vi "To Value.vi"(8 "error in (no error)":errorcluster, 10 "PV Data in":refnum<class "PV Data.lvclass">, 11 "NT Scalar (Numeric) in":refnum<class "NT Scalar (Numeric).lvclass">) -> (0 "error out":errorcluster, 2 "PV Data out":refnum<class "PV Data.lvclass">, 3 "NT Scalar (Numeric) out":refnum<class "NT Scalar (Numeric).lvclass">)   [LabVIEW 2020, in "PV Access.lvlib" / "PV Data.lvlib" / "NT Scalar (Numeric).lvclass"]
uses:
  NT Scalar (Numeric).lvclass
  NT Scalar (Numeric).lvclass/NT Scalar (Numeric).ctl
  PV Data/PV Data.lvclass
  PV Data/Write Field (Variant).vi
  NT Scalar/NT Scalar.lvclass
  PV Data/Write Field (String).vi
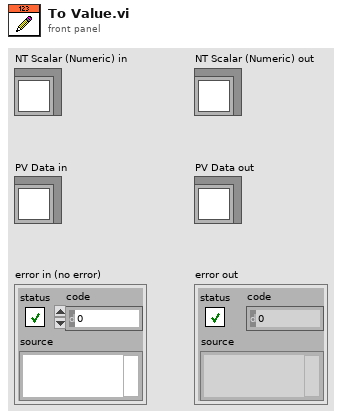
[diagram p1: front panel]
types:
  T1 = typedef "PV Access.lvlib/PV Data.lvlib/Alarm Limits.ctl" = cluster{"Active":bool, "Low Alarm Limit":variant, "Low Warning Limit":variant, "High Warning Limit":variant, "High Alarm Limit":variant, "Low Alarm Severity":T2, "Low Warning Severity":T2, "High Warning Severity ":T2, "High Alarm Severity":T2, "Hysteresis":dbl}
  T2 = typedef "PV Access.lvlib/PV Data.lvlib/Alarm Severity.ctl" = enum32{"no", "minor", "major", "record", "invalid", "undefined", ""}
  T3 = typedef "PV Access.lvlib/PV Data.lvlib/Display Form.ctl" = enum32{"Default", "String", "Binary", "Decimal", "Hex", "Exponential", "Engineering"}
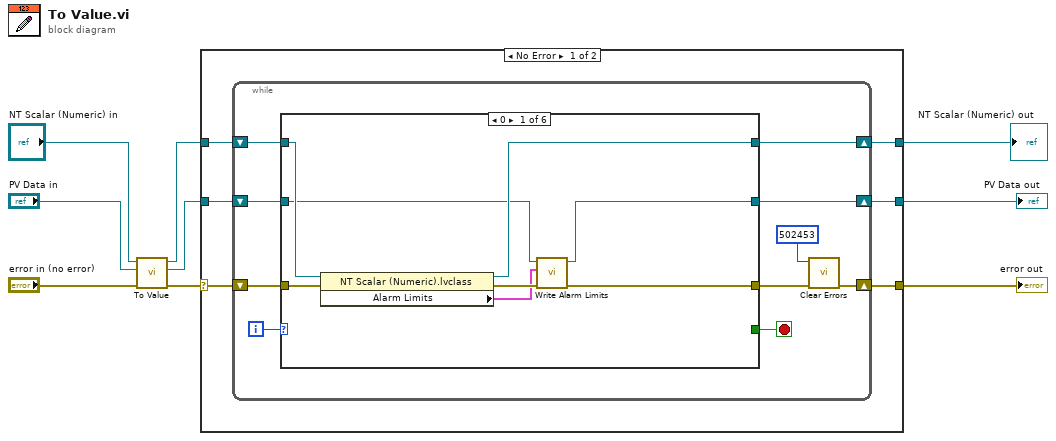
[diagram p0: block diagram]
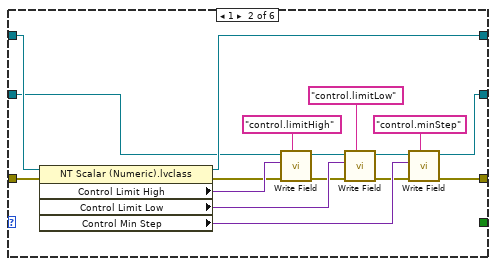
[diagram p2: hidden frame]
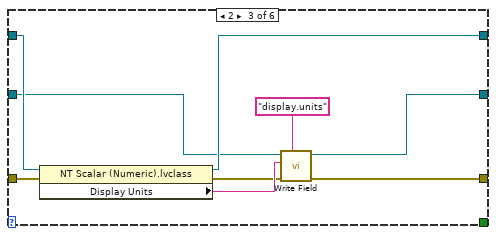
[diagram p3: hidden frame]
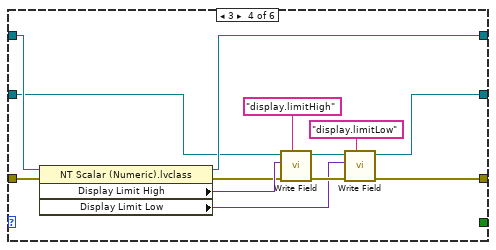
[diagram p4: hidden frame]
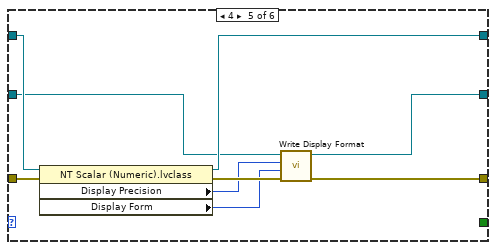
[diagram p5: hidden frame]
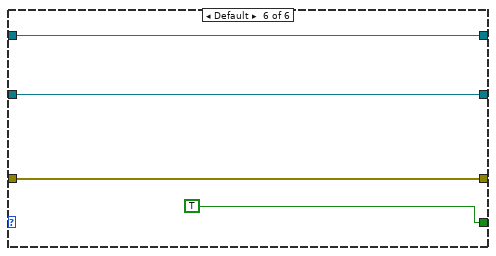
[diagram p6: hidden frame]
diagram:
  n1 = call-parent "To Value.vi"("error in (no error)"="error in (no error)", "PV Data in"="PV Data in", "NT Scalar in"="NT Scalar (Numeric) in") -> ("error out"=w5:errorcluster, "PV Data out"=w1:refnum<class "PV Data.lvclass">, "NT Scalar out"=w2:refnum<class "NT Scalar (Numeric).lvclass">)  [unwired: 6 in]
  n2 = case shown="No Error" w5 {
    selector: w5 -> [w15 w88]
    tunnel: [w12 w88] -> w7
    tunnel: [w10 w87] -> w9
    tunnel: w2 -> [w14 w87]
    tunnel: w1 -> [w13 w86]
    tunnel: [w11 w86] -> w8
    frame No Error {
      n3 = while {
        shift-right: [w19] -> w12
        shift-left: w15 -> [w24]
        shift-right: [w18] -> w11
        shift-left: w13 -> [w23]
        shift-right: [w17] -> w10
        shift-left: w14 -> [w22]
        i -> [w25]
        stop <- w16 stop-if-true
        n4 = case shown="0" w25 {
          tunnel: w24 -> [w33 w50 w59 w72 w81 w84]
          tunnel: w23 -> [w28 w39 w51 w62 w78 w83]
          tunnel: w22 -> [w32 w49 w58 w71 w80 w82]
          tunnel: [w26 w37 w54 w60 w76 w84] -> w20
          tunnel: [w27 w38 w55 w61 w77 w83] -> w18
          tunnel: [w31 w48 w57 w70 w79 w82] -> w17
          tunnel: [_ _ _ _ _ TRUE] -> w16
          frame 0 {
            n5 = property class="NT Scalar (Numeric).lvclass"(reference=w32, error in=w33) -> (reference out=w31:refnum<class "NT Scalar (Numeric).lvclass">, error out=w30:errorcluster, "Alarm Limits"=w29:T1)
            n6 = call "Write Alarm Limits.vi"("error in"=w30, "Alarm Limits"=w29, "PV Data in"=w28) -> ("error out"=w26:errorcluster, "PV Data out"=w27:refnum<class "PV Data.lvclass">)  [unwired: 7 in]
          }
          frame 1 {
            n7 = property class="NT Scalar (Numeric).lvclass"(reference=w49, error in=w50) -> (reference out=w48:refnum<class "NT Scalar (Numeric).lvclass">, error out=w44:errorcluster, "Control Limit High"=w47:variant, "Control Limit Low"=w46:variant, "Control Min Step"=w45:variant)
            n8 = call-poly "Write Field.vi"("field name"="control.limitHigh", "error in (no error)"=w44, "value in"=w47, "PV Data in"=w39) -> ("error out"=w43:errorcluster, "PV Data out"=w40:refnum<class "PV Data.lvclass">)  [unwired: 5 in, 1 out]
            n9 = call-poly "Write Field.vi"("field name"="control.limitLow", "error in (no error)"=w43, "value in"=w46, "PV Data in"=w40) -> ("error out"=w42:errorcluster, "PV Data out"=w41:refnum<class "PV Data.lvclass">)  [unwired: 5 in, 1 out]
            n10 = call-poly "Write Field.vi"("field name"="control.minStep", "error in (no error)"=w42, "value in"=w45, "PV Data in"=w41) -> ("error out"=w37:errorcluster, "PV Data out"=w38:refnum<class "PV Data.lvclass">)  [unwired: 5 in, 1 out]
          }
          frame 2 {
            n11 = property class="NT Scalar (Numeric).lvclass"(reference=w58, error in=w59) -> (reference out=w57:refnum<class "NT Scalar (Numeric).lvclass">, error out=w52:errorcluster, "Display Units"=w53:string)
            n12 = call-poly "Write Field.vi"("field name"="display.units", "error in"=w52, "value"=w53, "PV Data in"=w51) -> ("error out"=w54:errorcluster, "PV Data out"=w55:refnum<class "PV Data.lvclass">)  [unwired: 5 in, 1 out]
          }
          frame 3 {
            n13 = property class="NT Scalar (Numeric).lvclass"(reference=w71, error in=w72) -> (reference out=w70:refnum<class "NT Scalar (Numeric).lvclass">, error out=w63:errorcluster, "Display Limit High"=w65:variant, "Display Limit Low"=w64:variant)
            n14 = call-poly "Write Field.vi"("field name"="display.limitHigh", "error in (no error)"=w63, "value in"=w65, "PV Data in"=w62) -> ("error out"=w66:errorcluster, "PV Data out"=w67:refnum<class "PV Data.lvclass">)  [unwired: 5 in, 1 out]
            n15 = call-poly "Write Field.vi"("field name"="display.limitLow", "error in (no error)"=w66, "value in"=w64, "PV Data in"=w67) -> ("error out"=w60:errorcluster, "PV Data out"=w61:refnum<class "PV Data.lvclass">)  [unwired: 5 in, 1 out]
          }
          frame 4 {
            n16 = property class="NT Scalar (Numeric).lvclass"(reference=w80, error in=w81) -> (reference out=w79:refnum<class "NT Scalar (Numeric).lvclass">, error out=w75:errorcluster, "Display Precision"=w74:i32, "Display Form"=w73:T3)
            n17 = call "Write Display Format.vi"("error in"=w75, "form"=w73, "precision"=w74, "PV Data in"=w78) -> ("error out"=w76:errorcluster, "PV Data out"=w77:refnum<class "PV Data.lvclass">)  [unwired: 6 in]
          }
          frame Default {
          }
        }
        n18 = call <vilib>:"Clear Errors.vi"("error in (no error)"=w20, "specific error code to clear (0: all)"=502453) -> ("error out"=w19:errorcluster)  [unwired: 4 in, 1 out]
      }
    }
    frame Error {
    }
  }
  "error out" <- w7
  "NT Scalar (Numeric) out" <- w9
  "PV Data out" <- w8
